vi "SL TAGS Setup Tags.vi"(8 "error in (no error)":errorcluster, 9 "Set  Properties? (F)":bool, 11 "EEISysLink in":refnum<class "EEISysLink.lvclass">) -> (0 "error out":errorcluster, 3 "EEISysLink out":refnum<class "EEISysLink.lvclass">)   [LabVIEW 2017, in "EEISysLink.lvclass"]
doc: "Will update relevant non-value class tags to the SystemLink server. Currently this updates \"Collect Aggregates\" and properties.\n\nNote: to create class tags use the open tag method. \n\nJames Tillett P.E.\nEndeavor Engineering\nwww.endeavoreng.com"
uses:
  EEISysLink.lvclass
  EEISysLink.lvclass/EEISysLink.ctl
  <vilib>/Skyline/Tag/Wrapper/Wrapper_class/NI Skyline Tag.lvclass
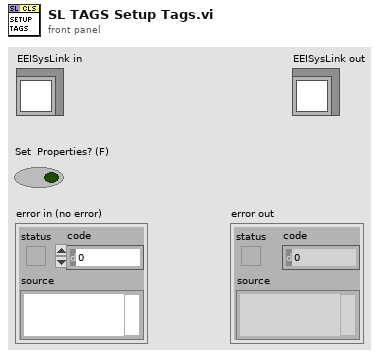
[diagram p1: front panel]
types:
  T1 = typedef "EEISysLink.lvclass/SL Tag.ctl" = cluster{"Class Properties":T2, "SL Tag":refnum<class "NI Skyline Tag.lvclass">, "SystemLink Cluster":T7, "Class Value":variant}
  T2 = typedef "EEISysLink.lvclass/SL Tag Properties.ctl" = cluster{"Class Data Type":T3, "Name":string, "Description":string, "Interpolation Method":T4, "Unit of Measure":T5, "Maximum Interpolation":string, "Role":T6}
  T3 = typedef "EEISysLink.lvclass/SL Tag Data Type.ctl" = enum16{"Double", "Integer", "String", "Boolean", "Waveform"}
  T4 = typedef "EEISysLink.lvclass/SL Tag Interpolation Method.ctl" = enum16{"linear", "pilinear", "step"}
  T5 = typedef "EEISysLink.lvclass/SL Tag Unit of Measure.ctl" = enum16{"no units", "Second", "Hour", "Minute", "Day", "Year", "Month", "Week", "Foot", "Yard", "Meter", "Centimeter", "Inch", "Mile", "Nautical Mile", "Miles per Hour", "Meters per second", "Square meter", "Cubic meter", "Cubic centimeter", "Cubic inch", "Liter", "Gallon", "Gallons dry US", "Gallon UK", "Percent", "Revolutions per minute", "Revolution", "Degree angle", "Astronomical Unit", "Atom", "Atomic mass", "Bar", "Byte", "C (speed of light)", "Curie", "Decibel", "Electron Volt", "Ounce", "Knot", "G", "Grade", "Are", "Hectare", "Faraday", "Franklin", "Gilbert", "Erg", "Lambert", "Maxwell", "Gauss", "Electron mass", "Kilogram force", "Pound force", "Rad", "Centiradian", "Sphere", "Mach", "Fluid Ounces", "Fluid Ounces UK", "Fahrenheit", "Celsius", "Kelvin", "Rankine", "Gram", "Kilogram", "Pound", "Short/US Ton", "Long/UK ton", "Metric ton", "Mole", "Pounds per square inch", "Inches water column", "Torr", "Millitorr", "Millimeter mercury", "Inches mercury", "Bar (2)", "Atmosphere", "Pascal", "Watt", "kiloWatt", "Horsepower", "Kilowatt Hour", "British thermal units", "Millions of BTU", "Ampere", "Candela", "Radian", "Steradian", "Bit", "Hertz", "Newton", "Joule", "Coulomb", "Volt", "Farad", "Ohm", "Siemens", "Weber", "Tesla", "Henry", "Lumen", "Lux", "Becqueral", "Gray", "Sievert", "Katal", "Angstrom", "Light Year", "Parsec", "Point", "Pixel", "Dyne", "Kilogram force (2)", "Pound force (2)", "Rem", "Rutherford", "Roentgen"}
  T6 = typedef "EEISysLink.lvclass/SL Tag Type.ctl" = enum16{"All", "Supervisor", "Worker"}
  T7 = typedef "NI Skyline Tag.lvlib/Tag Cluster.ctl" = cluster{"Path":string, "Data Type":T8, "Value":variant, "Time Stamp":timestamp}
  T8 = typedef "NI Skyline Tag.lvlib/DataType.ctl" = enum32{"Double", "Integer", "String"}
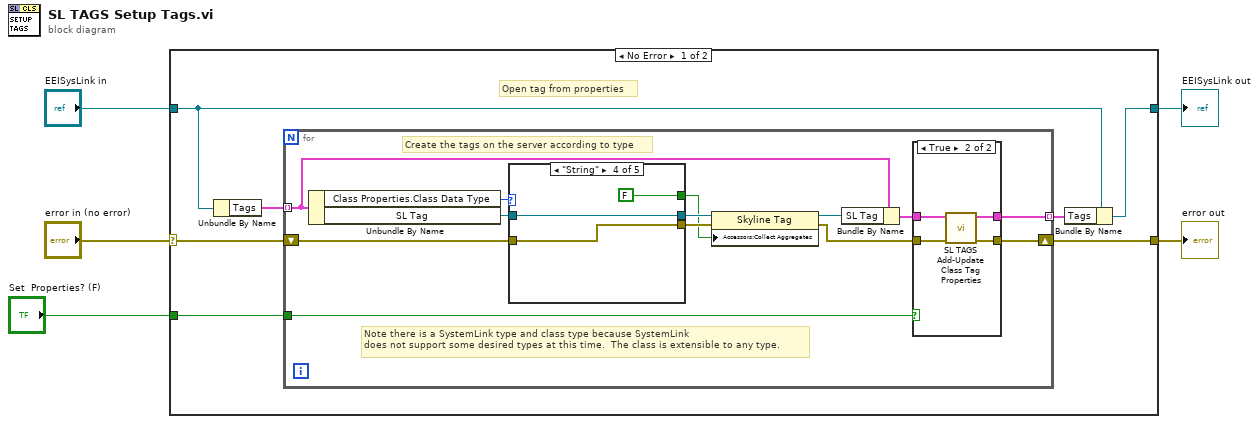
[diagram p0: block diagram]
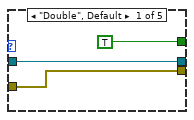
[diagram p3: hidden frame]
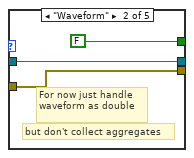
[diagram p4: hidden frame]
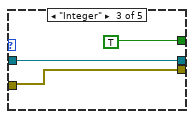
[diagram p5: hidden frame]
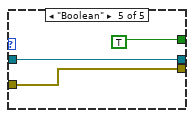
[diagram p6: hidden frame]
diagram:
  n1 = case shown="No Error" "error in (no error)" {
    selector: "error in (no error)" -> [w12 w48]
    tunnel: [w6 w48] -> w4
    tunnel: [w8 w47] -> w2
    tunnel: "EEISysLink in" -> [w9 w47]
    tunnel: "Set  Properties? (F)" -> [w10 _]
    frame No Error {
      # "Open tag from properties"
      n2 = Unbundle By Name(w9) -> ("Tags"=w11:T1[])
      n3 = for {
        tunnel: w11 -> [w22] mode=indexing
        shift-right: [w19] -> w6
        shift-left: w12 -> [w23]
        tunnel: w10 -> [w20]
        tunnel: [w18] -> w7 mode=indexing
        # "Note there is a SystemLink type and class type because SystemLink\ndoes not support some desired types at this time.  The class is extensible to any type."
        # "Create the tags on the server according to type"
        n4 = Unbundle By Name(w22) -> ("Class Properties.Class Data Type"=w24:T3, "SL Tag"=w25:refnum<class "NI Skyline Tag.lvclass">)
        n5 = case shown="\"String\"" w24 {
          tunnel: w25 -> [w34 w37 w40 w43 w46]
          tunnel: [w34 w37 w40 w43 w46] -> w17
          tunnel: [w33 w36 w39 w42 w45] -> w15
          tunnel: w23 -> [w33 w36 w39 w42 w45]
          tunnel: [TRUE ("Collect Aggregates") FALSE ("Collect Aggregates") TRUE ("Collect Aggregates") FALSE ("Collect Aggregates") TRUE ("Collect Aggregates")] -> w14
          frame "Double", Default {
          }
          frame "Waveform" {
            # "but don't collect aggregates"
            # "For now just handle \nwaveform as double"
          }
          frame "Integer" {
          }
          frame "String" {
          }
          frame "Boolean" {
          }
        }
        n6 = property class="Skyline Tag"(reference=w17, error in=w15, "Accessors:Collect Aggregates"=w14) -> (reference out=w16:refnum<class "NI Skyline Tag.lvclass">, error out=w13:errorcluster)
        n7 = Bundle By Name(cluster=w22, "SL Tag"=w16) -> (w21:T1)
        n8 = case shown="True" w20 {
          tunnel: w21 -> [w26 w30]
          tunnel: w13 -> [w27 w31]
          tunnel: [w27 w28] -> w19
          tunnel: [w26 w29] -> w18
          frame False {
          }
          frame True {
            n9 = call "SL TAGS Add-Update Class Tag Properties.vi"("error in (no error)"=w31, "Tag In"=w30) -> ("error out"=w28:errorcluster, "Tag Ref Out"=w29:T1)  [unwired: 8 in]
          }
        }
      }
      n10 = Bundle By Name(cluster=w9, "Tags"=w7) -> (w8:refnum<class "EEISysLink.lvclass">)
    }
    frame Error {
    }
  }
  "error out" <- w4
  "EEISysLink out" <- w2
